vi "MDPtr Pack Memory.vi"(6 "DT":T1, 7 "Copies Count(1)":i32=1, 9 "String Attribute":string, 10 "error in (no error)":errorcluster, 11 "String":string) -> (2 "error out":errorcluster, 3 "HexStrPtr":T2)   [LabVIEW 2017, in "MDPtr.lvlib"]
uses:
  MDPtr.lvlib
  MDPtr TypeDef/MDPtr.ctl
  <vilib>/Utility/Data Type/Type Definitions/Data Type.ctl
  MDPtr TypeDef/MDPtr DataFrame-Memory.ctl
  MDPtr TypeDef/MDPtr DataFrame-Common.ctl
  _MDPtrMgr/MDPtrMgr.lvclass
  <vilib>/Utility/Data Type/NI_Data Type.lvlib
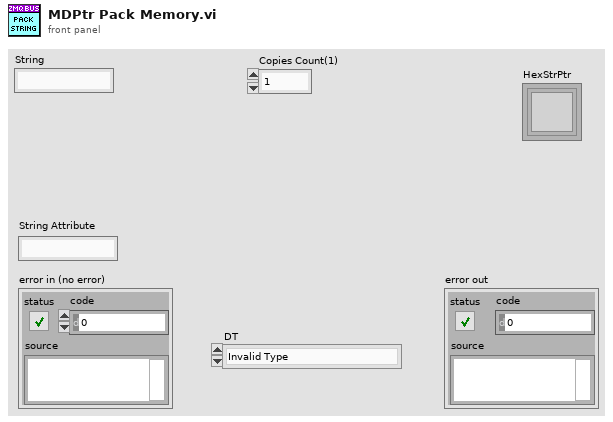
[diagram p1: front panel]
types:
  T1 = typedef "NI_Data Type.lvlib/Data Type.ctl" = enum8{"Invalid Type", "Void", "I8", "I16", "I32", "I64", "U8", "U16", "U32", "U64", "Single Float", "Double Float", "Extended Float", "Single Complex", "Double Complex", "Extended Complex", "Enum U8", "Enum U16", "Enum U32", "Enum U64", "Single Float With Unit", "Double Float With Unit", "Extended Float With Unit", "Single Complex with Unit", "Double Complex with Unit", "Extended Complex with Unit", "Boolean", "String", "Path", "Picture", "Tag", "Array", "Cluster", "Variant", "LV Variant", "Waveform", "Timestamp", "Digital Waveform", "Digital Data", "ExpressData", "Refnum", "External Data", "VI", "Poly VI", "LabVIEW Class Instance", "Fixed Point"}
  T2 = typedef "MDPtr.lvlib/MDPtr.ctl" = refnum<k1>
  T3 = typedef "MDPtr.lvlib/MDPtr DataFrame-Memory.ctl" = cluster{"Common":T4, "DVR":refnum<data-value>}
  T4 = typedef "MDPtr.lvlib/MDPtr DataFrame-Common.ctl" = cluster{"Data Type":T1, "Copy Count":i32, "String Attribute":string}
  T5 = typedef "MDPtr.lvlib/Def-MDPtrQueue.ctl" = refnum<queue>
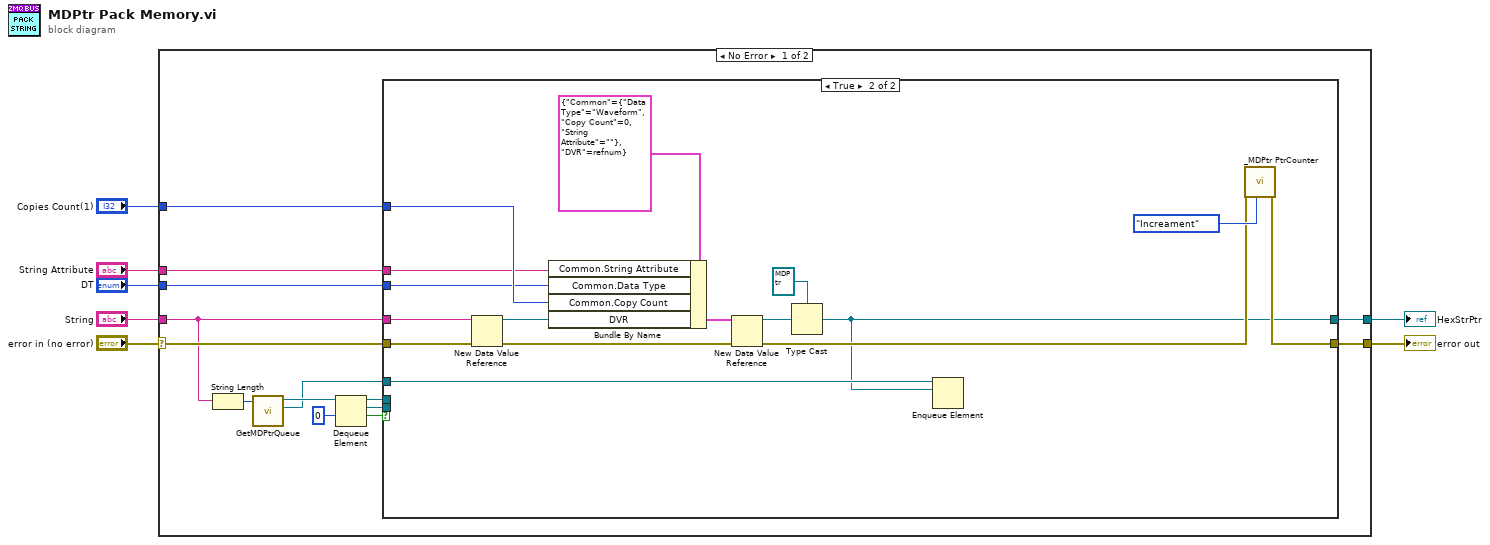
[diagram p0: block diagram]
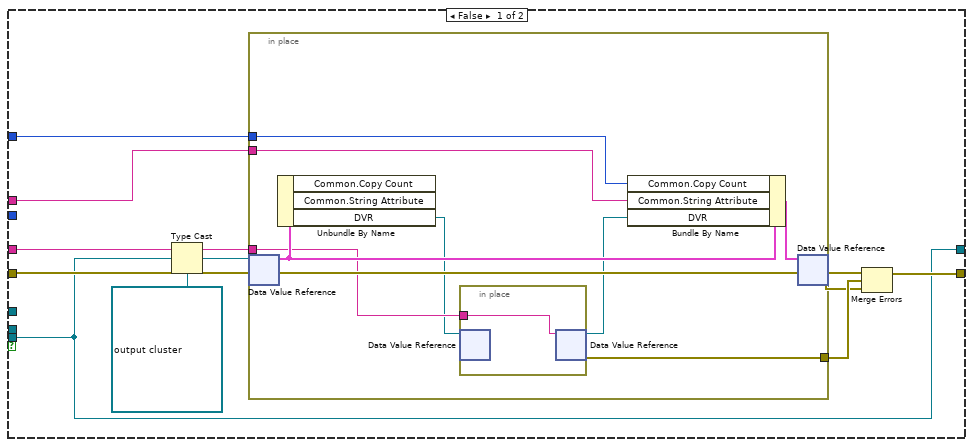
[diagram p2: hidden frame]
diagram:
  n1 = case shown="No Error" "error in (no error)" {
    selector: "error in (no error)" -> [w21 w57]
    tunnel: [w20 w57] -> w6
    tunnel: "String" -> [w13 _]
    tunnel: [w19 _] -> w4
    tunnel: "Copies Count(1)" -> [w18 _]
    tunnel: "String Attribute" -> [w17 _]
    tunnel: "DT" -> [w8 _]
    frame No Error {
      n2 = String Length(string=w13) -> (length=w14:i32)
      n3 = call "GetMDPtrQueue.vi"("MemoryLength"=w14) -> ("Total MDPtrQueue"=w9:T5, "MDPtrQueue"=w15:T5)  [unwired: 8 in, 1 out]
      n4 = Dequeue Element(queue=w15, timeout in ms (-1)=0) -> (queue out=w12:T5, element=w10:T2, timed out?=w11:bool)  [unwired: 1 in, 1 out]
      n5 = case shown="True" w11 {
        tunnel: w21 -> [w27 w55]
        tunnel: [w26 w51] -> w20
        tunnel: [w22 w42] -> w19
        tunnel: w18 -> [w24 w48]
        tunnel: w17 -> [w23 w45]
        tunnel: w13 -> [w25 w44]
        tunnel: w12 -> [_ _]
        tunnel: w10 -> [w22 _]
        tunnel: w9 -> [_ w43]
        tunnel: w8 -> [_ w41]
        frame False {
          n6 = Type Cast(type=refnum<data-value> refnum ("data value reference"), x=w22) -> (*(type *) &x=w31:refnum<data-value>)
          n7 = in-place {
            in-place-border: [w37] -> w29
            in-place-border: w25 -> [w36]
            in-place-border: w23 -> [w35]
            in-place-border: w24 -> [w34]
            n8 = in-place-dvr #1(w31) -> (w39:T3)  [unwired: 1 out]
            n9 = Unbundle By Name(w39) -> ("DVR"=w33:refnum<data-value>)  [unwired: 2 out]
            n10 = in-place {
              in-place-border: w36 -> [w40]
              n11 = in-place-dvr #2(w33) -> ()  [unwired: 2 out]
              n12 = in-place-dvr #2(w40) -> (w32:refnum<data-value>, w37:errorcluster)
            }
            n13 = Bundle By Name(cluster=w39, "Common.Copy Count"=w34, "Common.String Attribute"=w35, "DVR"=w32) -> (w38:T3)
            n14 = in-place-dvr #1(w38) -> (w28:errorcluster)  [unwired: 1 out]
          }
          n15 = Merge Errors(w27, w29, w28) -> (w26:errorcluster)
        }
        frame True {
          n16 = New Data Value Reference(data value=w44, error in=w55) -> (data value reference=w49:refnum<data-value>, error out=w54:errorcluster)
          n17 = Bundle By Name(cluster=T3 {"Common"={"Data Type"=enum."Waveform", "Copy Count"=0, "String Attribute"=""}, "DVR"=refnum} ("DataFrame-String"), "Common.String Attribute"=w45, "Common.Data Type"=w41, "Common.Copy Count"=w48, "DVR"=w49) -> (w56:T3)
          n18 = New Data Value Reference(data value=w56, error in=w54) -> (data value reference=w50:refnum<data-value>, error out=w52:errorcluster)
          n19 = Type Cast(type=T2 refnum ("MDPtr"), x=w50) -> (*(type *) &x=w42:T2)
          n20 = Enqueue Element(queue=w43, element=w42) -> ()  [unwired: 2 in, 3 out]
          n21 = call "_MDPtr PtrCounter.vi"("Oper(Get)"=enum16{"GET", "Increament", "decreament"}."Increament", "error in (no error)"=w52) -> ("error out"=w51:errorcluster)  [unwired: 8 in, 1 out]
        }
      }
    }
    frame Error {
    }
  }
  "HexStrPtr" <- w4
  "error out" <- w6
